vi "loadDataNodeBegin.vi"(8 "error in (no error)":errorcluster, 10 "XML Refnum in":refnum<file>, 11 "Packet in":refnum<class "Packet.lvclass">) -> (0 "error out":errorcluster, 2 "XML Refnum out":refnum<file>, 3 "Packet out":refnum<class "Packet.lvclass">)   [LabVIEW 2013, in "Packet.lvclass"]
doc: "Part of the file loading process. Occurs at the beginning of a node being loaded. Loads the common xceDataNode data name and description."
uses:
  Packet.lvclass
  xCE/xceNode/xceNode.lvclass
  XML Parser/XML Parser.lvclass
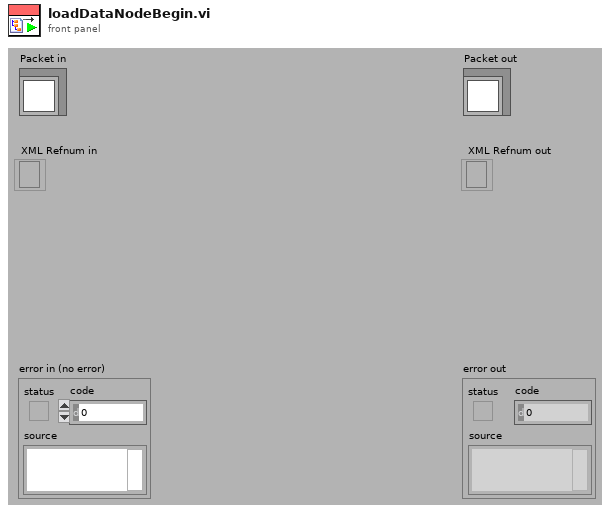
[diagram p1: front panel]
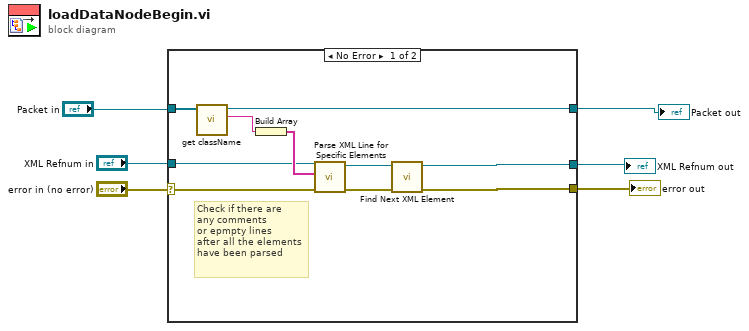
[diagram p0: block diagram]
diagram:
  n1 = case shown="No Error" "error in (no error)" {
    selector: "error in (no error)" -> [w11 w19]
    tunnel: [w7 w19] -> w3
    tunnel: [w12 w18] -> w5
    tunnel: "Packet in" -> [w16 w18]
    tunnel: "XML Refnum in" -> [w13 w17]
    tunnel: [w9 w17] -> w4
    frame No Error {
      # "Check if there are\nany comments \nor epmpty lines\nafter all the elements\nhave been parsed"
      n2 = call "get className.vi"("xceNode in"=w16) -> ("Class name"=w14:string, "xceNode out"=w12:refnum<class "Packet.lvclass">)  [unwired: 8 in, 1 out]
      n3 = Build Array(w14) -> (w15:string[])
      n4 = call "Parse XML Line for Specific Elements.vi"("error in (no error)"=w11, "Elements"=w15, "XML Refnum in"=w13) -> ("error out"=w8:errorcluster, "XML Refnum out"=w10:refnum<file>)  [unwired: 4 in, 3 out]
      n5 = call "Find Next XML Element.vi"("error in (no error)"=w8, "XML Fine In"=w10) -> ("error out"=w7:errorcluster, "XML Fine Out"=w9:refnum<file>)  [unwired: 7 in, 1 out]
    }
    frame Error {
    }
  }
  "error out" <- w3
  "Packet out" <- w5
  "XML Refnum out" <- w4
